vi "add line.vi"(8 "error in":errorcluster, 10 "Line":T1, 11 "TDMS datalogger configuration in":refnum<class "TDMS datalogger configuration.lvclass">) -> (0 "error out":errorcluster, 2 "Line Index":i32, 3 "TDMS datalogger configuration out":refnum<class "TDMS datalogger configuration.lvclass">)   [LabVIEW 2015, in "TDMS datalogger configuration.lvclass"]
uses:
  TDMS datalogger configuration.lvclass
  <vilib>/NI/Tag Bus Module Framework/channel/TBM channel.lvclass
  TDMS datalogger configuration.lvclass/TDMS datalogger configuration.ctl
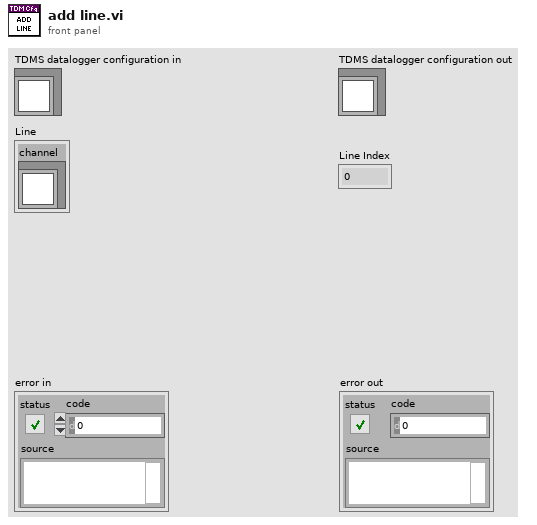
[diagram p1: front panel]
types:
  T1 = cluster{"channel":refnum<class "TBM channel.lvclass">}
  T2 = cluster{"channel":refnum<class "TBM channel.lvclass">}[]
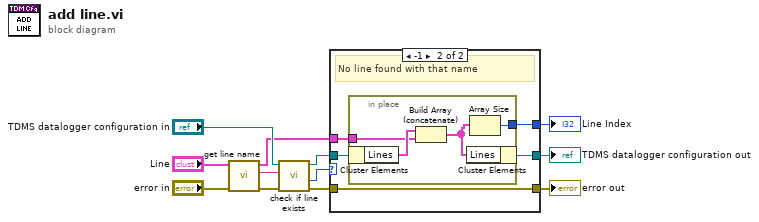
[diagram p0: block diagram]
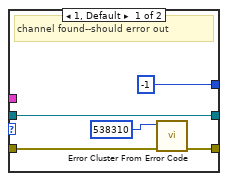
[diagram p2: hidden frame]
diagram:
  n1 = call "get line name.vi"("error in"="error in", "line in"="Line") -> ("error out"=w10:errorcluster, "Name"=w9:string, "line out"=w5:T1)  [unwired: 7 in]
  n2 = call "check if line exists.vi"("error in"=w10, "Name to Locate"=w9, "TDMS datalogger configuration"="TDMS datalogger configuration in") -> ("error out"=w6:errorcluster, "Index"=w7:i32, "TDMS datalogger configuration"=w1:refnum<class "TDMS datalogger configuration.lvclass">)  [unwired: 4 in, 2 out]
  n3 = case shown="-1" w7 {
    tunnel: [w17 w21] -> w4
    tunnel: w6 -> [w15 w21]
    tunnel: w1 -> [w14 w20]
    tunnel: w5 -> [_ w22]
    tunnel: [w14 w19] -> w3
    tunnel: [-1 w18] -> w2
    frame 1, Default {
      # "channel found--should error out"
      n4 = call <vilib>:"Error Cluster From Error Code.vi"("error in (no error)"=w15, "error code (0)"=538310) -> ("error out"=w17:errorcluster)  [unwired: 7 in]
    }
    frame -1 {
      # "No line found with that name"
      n5 = in-place {
        in-place-border: w22 -> [w25]
        in-place-border: [w23] -> w18
        n6 = in-place-cluster #1(w20) -> ("Lines"=w26:T2)
        n7 = Build Array (concatenate)(w26, w25) -> (w24:T2)
        n8 = in-place-cluster #1("Lines"=w24) -> (w19:refnum<class "TDMS datalogger configuration.lvclass">)
        n9 = Array Size(array=w24) -> (size(s)=w23:i32)
      }
    }
  }
  "error out" <- w4
  "TDMS datalogger configuration out" <- w3
  "Line Index" <- w2
